vi "CreateWO-CreateWordDocument.vi"(7 "error in":errorcluster, 10 "Input Word Cluster":T1={"Cert Yes or No"="Testing Cert", "Date Created"="Date", "Inspect"="Inspect", "Lot Number"="Lot Number", "Manufacturer"="Manufactuer", "Customer"="Customer", "Start Date"="Due Date", "Date Required"="Date Required", "Part Number"="Part Number", "Part Description"="Part Descritption", "Quantity"="50", "Work Order"="Work Order", "Sales Order"="Work Order", "Shipper"="Shipper", "Special Instructions"="Shipper"}) -> (0 "error out":errorcluster, 2 "Word Doc Not Created":bool, 3 "Path for Outlook":path)   [LabVIEW 2013, in "ERP-CreateWorkOrder.lvclass"]
uses:
  ERP-CreateWorkOrder.lvclass
panel:
  in  "Word._Application":refnum<k7>
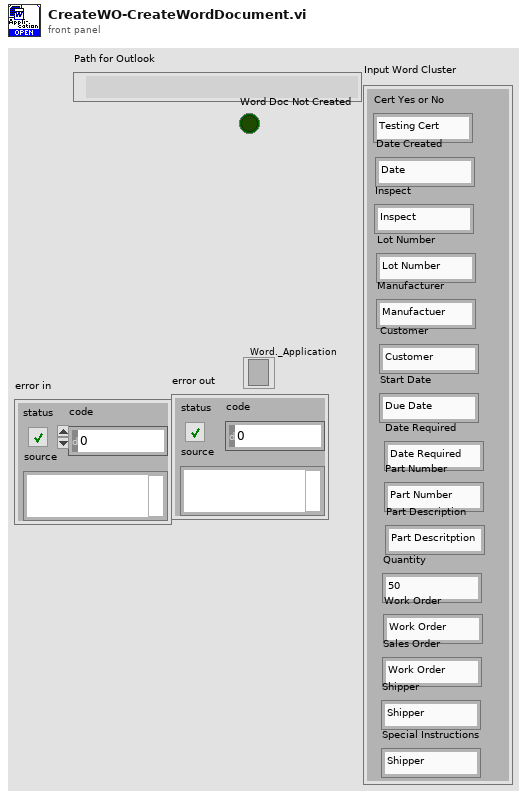
[diagram p1: front panel]
types:
  T1 = cluster{"Cert Yes or No":string, "Date Created":string, "Inspect":string, "Lot Number":string, "Manufacturer":string, "Customer":string, "Start Date":string, "Date Required":string, "Part Number":string, "Part Description":string, "Quantity":string, "Work Order":string, "Sales Order":string, "Shipper":string, "Special Instructions":string}
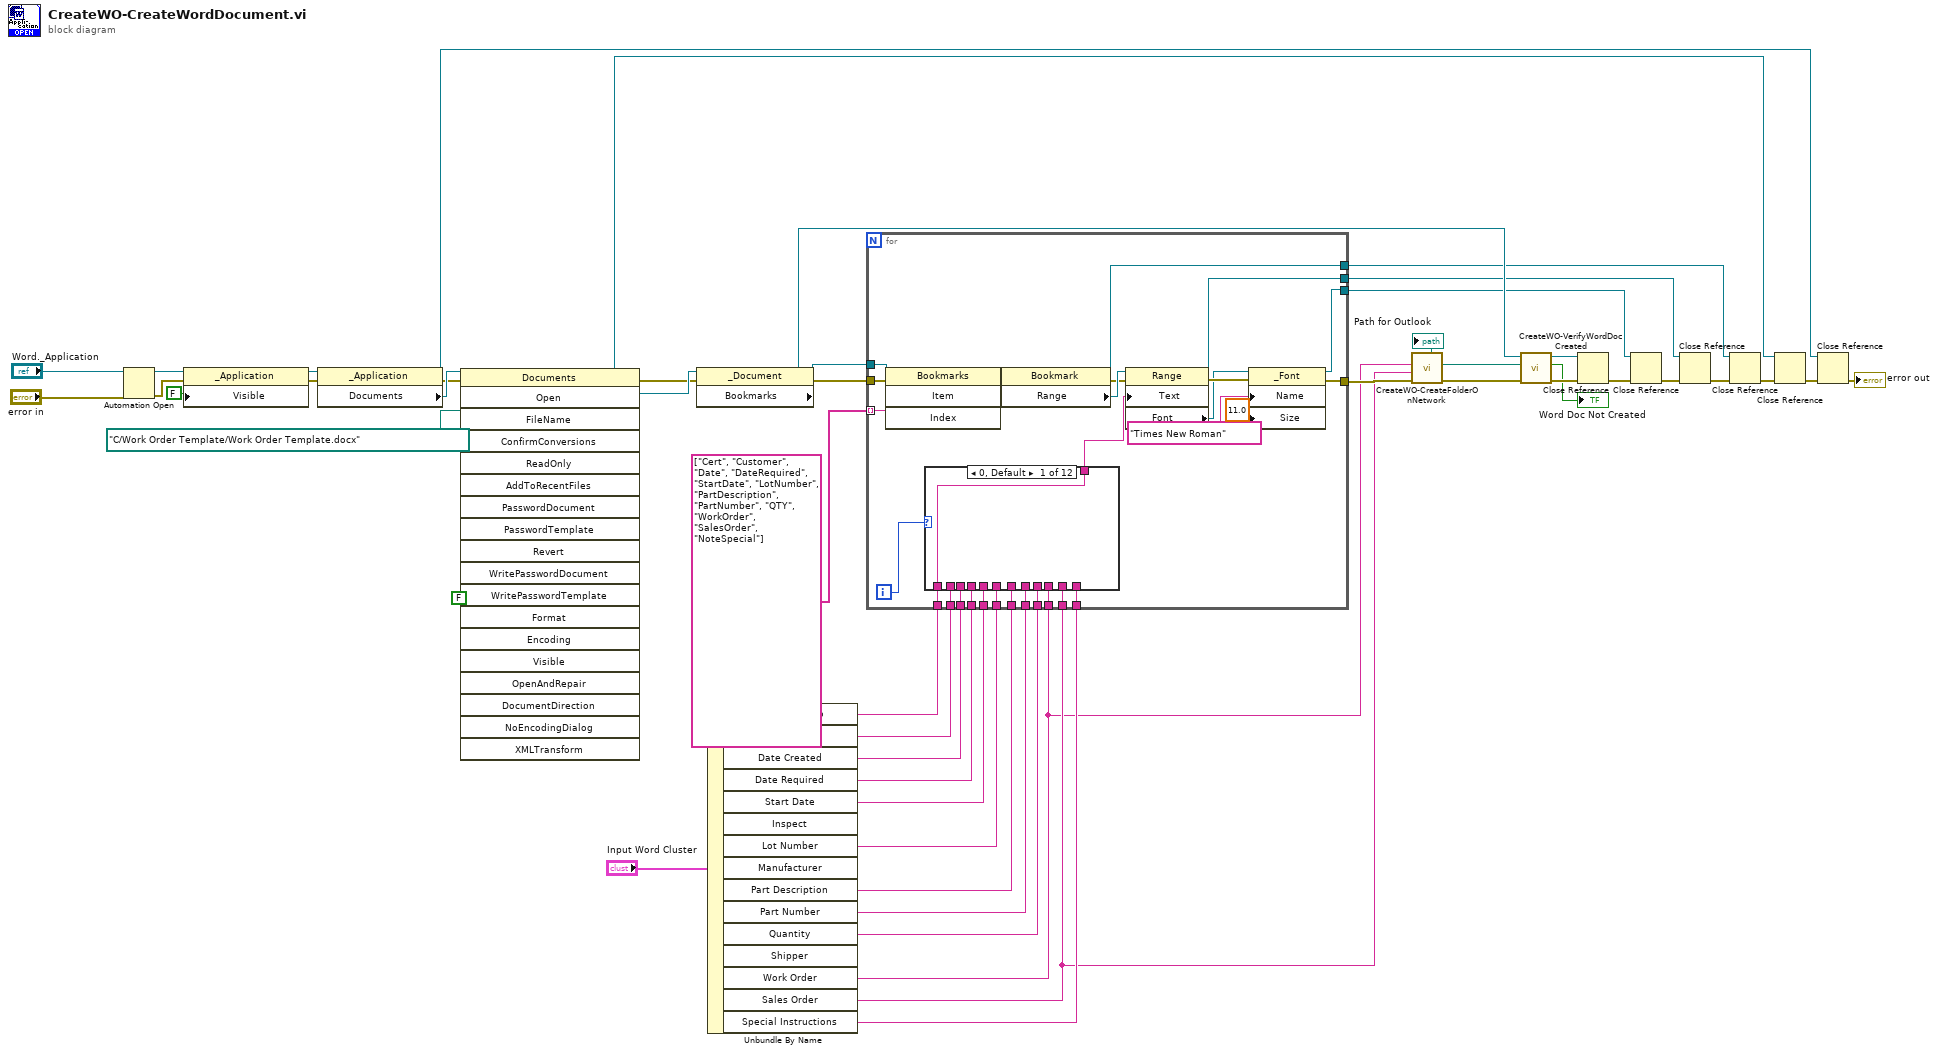
[diagram p0: block diagram]
diagram:
  n1 = Automation Open(error in (no error)="error in", Automation Refnum="Word._Application") -> (Automation Refnum=w42:refnum<k7>, error out=w36:errorcluster)  [unwired: 2 in]
  n2 = property class="_Application"(reference=w42, error in=w36, "Visible"=FALSE) -> (reference out=w41:refnum<k7>, error out=w40:errorcluster)
  n3 = property class="_Application"(reference=w41, error in=w40) -> (reference out=w37:refnum<k7>, error out=w47:errorcluster, "Documents"=w48:refnum<k7>)
  n4 = invoke class="Documents" method="Open"(reference=w48, error in=w47, "FileName"=path "C:/Work Order Template/Work Order Template.docx", "Visible"=FALSE) -> (reference out=w38:refnum<k7>, error out=w18:errorcluster, "Open"=w33:refnum<k7>)  [unwired: 15 in, 16 out]
  n5 = property class="_Document"(reference=w33, error in=w18) -> (reference out=w19:refnum<k7>, error out=w30:errorcluster, "Bookmarks"=w31:refnum<k7>)
  n6 = Unbundle By Name("Input Word Cluster") -> ("Cert Yes or No"=w29:string, "Customer"=w28:string, "Date Created"=w27:string, "Date Required"=w26:string, "Start Date"=w25:string, "Lot Number"=w24:string, "Part Description"=w23:string, "Part Number"=w22:string, "Quantity"=w21:string, "Work Order"=w6:string, "Sales Order"=w7:string, "Special Instructions"=w20:string)  [unwired: 3 out]
  n7 = for {
    tunnel: string[] ["Cert", "Customer", "Date", "DateRequired", "StartDate", "LotNumber", "PartDescription", "PartNumber", "QTY", "WorkOrder", "SalesOrder", "NoteSpecial"] -> [w75] mode=indexing
    tunnel: w31 -> [w74]
    tunnel: w30 -> [w73]
    tunnel: w29 -> [w69]
    tunnel: w28 -> [w67]
    tunnel: w27 -> [w66]
    tunnel: w26 -> [w65]
    tunnel: w25 -> [w64]
    tunnel: w24 -> [w63]
    tunnel: w23 -> [w62]
    tunnel: w22 -> [w61]
    tunnel: w21 -> [w60]
    tunnel: w6 -> [w59]
    tunnel: w7 -> [w58]
    tunnel: w20 -> [w57]
    tunnel: [w50] -> w8
    tunnel: [w56] -> w17
    tunnel: [w55] -> w15
    tunnel: [w49] -> w9
    i -> [w70]
    n8 = invoke class="Bookmarks" method="Item"(reference=w74, error in=w73, "Index"=w75) -> (error out=w76:errorcluster, "Item"=w77:refnum<k7>)  [unwired: 1 in, 2 out]
    n9 = case shown="0, Default" w70 {
      tunnel: [w78 w79 w80 w81 w82 w83 w84 w85 w86 w87 w88 w89] -> w68
      tunnel: w69 -> [w78 _ _ _ _ _ _ _ _ _ _ _]
      tunnel: w67 -> [_ w79 _ _ _ _ _ _ _ _ _ _]
      tunnel: w66 -> [_ _ w80 _ _ _ _ _ _ _ _ _]
      tunnel: w65 -> [_ _ _ w81 _ _ _ _ _ _ _ _]
      tunnel: w64 -> [_ _ _ _ w82 _ _ _ _ _ _ _]
      tunnel: w63 -> [_ _ _ _ _ w83 _ _ _ _ _ _]
      tunnel: w62 -> [_ _ _ _ _ _ w84 _ _ _ _ _]
      tunnel: w61 -> [_ _ _ _ _ _ _ w85 _ _ _ _]
      tunnel: w60 -> [_ _ _ _ _ _ _ _ w86 _ _ _]
      tunnel: w59 -> [_ _ _ _ _ _ _ _ _ w87 _ _]
      tunnel: w58 -> [_ _ _ _ _ _ _ _ _ _ w88 _]
      tunnel: w57 -> [_ _ _ _ _ _ _ _ _ _ _ w89]
      frame 0, Default {
      }
      frame 1 {
      }
      frame 2 {
      }
      frame 3 {
      }
      frame 4 {
      }
      frame 5 {
      }
      frame 6 {
      }
      frame 7 {
      }
      frame 8 {
      }
      frame 9 {
      }
      frame 10 {
      }
      frame 11 {
      }
    }
    n10 = property class="Bookmark"(reference=w77, error in=w76) -> (reference out=w55:refnum<k7>, error out=w71:errorcluster, "Range"=w72:refnum<k7>)
    n11 = property class="Range"(reference=w72, error in=w71, "Text"=w68) -> (reference out=w56:refnum<k7>, error out=w53:errorcluster, "Font"=w51:refnum<k7>)
    n12 = property class="_Font"(reference=w51, error in=w53, "Name"="Times New Roman", "Size"=sgl 11.0) -> (reference out=w49:refnum<k7>, error out=w50:errorcluster)
  }
  n13 = call "CreateWO-CreateFolderOnNetwork.vi"("error in (no error)"=w8, "Sales Order"=w7, "Work Order"=w6) -> ("error out"=w5:errorcluster, "Path for Saving the file"=w3:path, "Path for Outlook"=→"Path for Outlook":path)  [unwired: 4 in, 2 out]
  n14 = call "CreateWO-VerifyWordDocCreated.vi"("error in (no error)"=w5, "Path for Saving the file"=w3, "Automation Refnum in"=w19) -> ("error out"=w13:errorcluster, "Word Doc Not Created"=→"Word Doc Not Created":bool, "Automation Refnum out"=w12:refnum<k7>)  [unwired: 6 in]
  n15 = Close Reference(reference=w12, error in (no error)=w13) -> (error out=w10:errorcluster)
  n16 = Close Reference(reference=w9, error in (no error)=w10) -> (error out=w11:errorcluster)
  n17 = Close Reference(reference=w17, error in (no error)=w11) -> (error out=w16:errorcluster)
  n18 = Close Reference(reference=w15, error in (no error)=w16) -> (error out=w14:errorcluster)
  n19 = Close Reference(reference=w38, error in (no error)=w14) -> (error out=w45:errorcluster)
  n20 = Close Reference(reference=w37, error in (no error)=w45) -> (error out=→"error out":errorcluster)
